vi "Check Gate.vi"(8 "error in (no error)":errorcluster, 9 "timeout in ms (-1)":i32=-1, 11 "gate":T1) -> (0 "error out":errorcluster, 1 "timed out?":bool, 3 "gate out":T1)   [LabVIEW 2015, in "Gates.lvlib"]
doc: "Checks the gate and waits until it is opened or timeout occurred."
uses:
  Gates.lvlib
  Gate.ctl
  Gate Pass.ctl
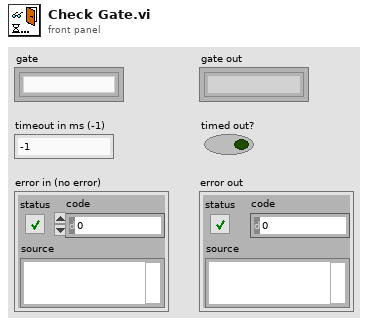
[diagram p1: front panel]
types:
  T1 = typedef "Gates.lvlib/Gate.ctl" = refnum<k1>
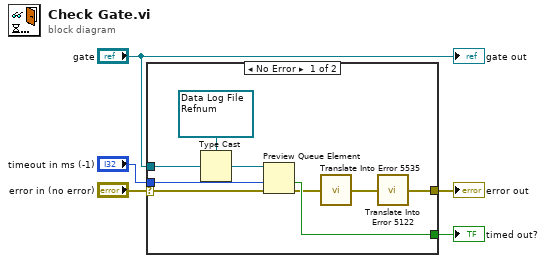
[diagram p0: block diagram]
diagram:
  n1 = case shown="No Error" "error in (no error)" {
    selector: "error in (no error)" -> [w12 w15]
    tunnel: [w6 w15] -> w4
    tunnel: "gate" -> [w14 _]
    tunnel: "timeout in ms (-1)" -> [w11 _]
    tunnel: [w10 _] -> w2
    frame No Error {
      w13 = refnum<queue> refnum items=["Gate Pass"] ("queue out")
      n2 = Type Cast(type=w13, x=w14) -> (*(type *) &x=w9:refnum<queue>)
      n3 = Preview Queue Element(queue=w9, timeout in ms (-1)=w11, error in (no error)=w12) -> (timed out?=w10:bool, error out=w7:errorcluster)  [unwired: 2 out]
      n4 = call "Translate Into Error 5535.vi"("error in (no error)"=w7) -> ("error out"=w8:errorcluster)  [unwired: 1 in]
      n5 = call "Translate Into Error 5122.vi"("error in (no error)"=w8) -> ("error out"=w6:errorcluster)  [unwired: 1 in]
    }
    frame Error {
    }
  }
  "error out" <- w4
  "timed out?" <- w2
  "gate out" <- "gate"
